vi "Read Status.vi"(8 "error in (no error)":errorcluster, 11 "Status in":refnum<class "Status.lvclass">) -> (0 "error out":errorcluster, 2 "Status":variant, 3 "Status out":refnum<class "Status.lvclass">)   [LabVIEW 2017, in "Message Interface.lvlib" / "Status.lvclass"]
uses:
  Status.lvclass
  Status.lvclass/Status.ctl
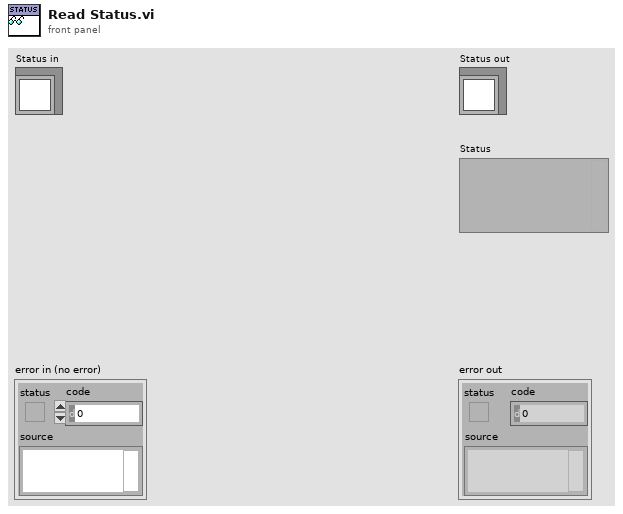
[diagram p1: front panel]
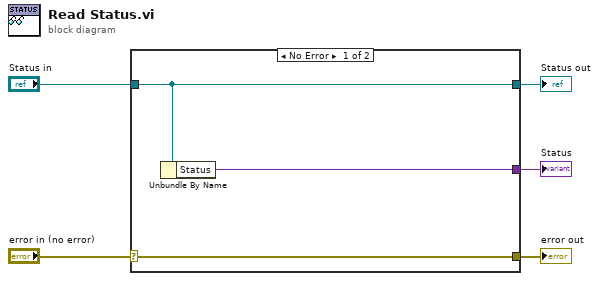
[diagram p0: block diagram]
diagram:
  n1 = case shown="No Error" "error in (no error)" {
    selector: "error in (no error)" -> [w8 w9]
    tunnel: [w8 w9] -> w4
    tunnel: [w7 w10] -> w2
    tunnel: "Status in" -> [w7 w10]
    tunnel: [w6 _] -> w1
    frame No Error {
      n2 = Unbundle By Name(w7) -> ("Status"=w6:variant)
    }
    frame Error {
    }
  }
  "error out" <- w4
  "Status out" <- w2
  "Status" <- w1
